vi "End experiment.vi"(7 "API Key":string, 8 "error in":errorcluster, 11 "Experiment ID":i32) -> (0 "error out":errorcluster)   [LabVIEW 2018]
uses:
  <vilib>/httpClient/PUTBuffer.vi
  <vilib>/httpClient/LabVIEWHTTPClient.lvlib
panel:
  out "Ended at response":string
  out "Server response debug panel":string
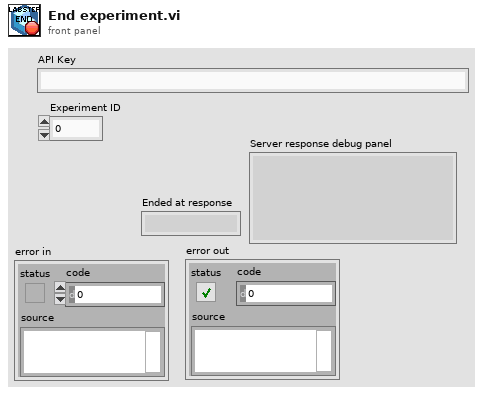
[diagram p1: front panel]
types:
  T1 = typedef "LabVIEWHTTPClient.lvlib/ClientHandle.ctl" = refnum<k1>
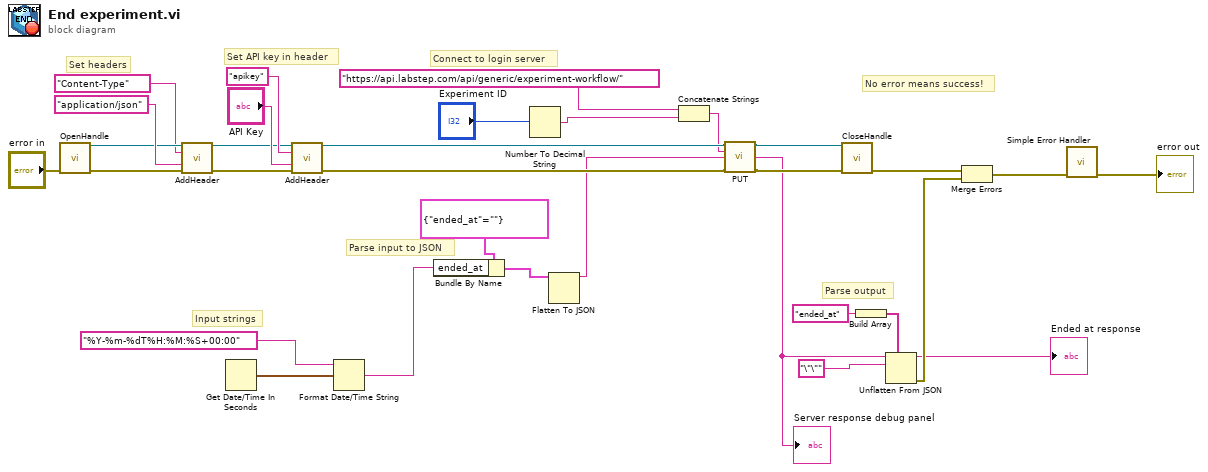
[diagram p0: block diagram]
diagram:
  # "No error means success!"
  # "Parse output"
  # "Set API key in header"
  # "Input strings"
  # "Set headers"
  # "Connect to login server"
  # "Parse input to JSON"
  n1 = call <vilib>:"OpenHandle.vi"("error in (no error)"="error in") -> ("client handle out"=w31:T1, "error out"=w30:errorcluster)  [unwired: 13 in]
  n2 = call <vilib>:"AddHeader.vi"("client handle"=w31, "header"="Content-Type", "value"="application/json", "error in (no error)"=w30) -> ("client handle out"=w22:T1, "error out"=w23:errorcluster)  [unwired: 10 in]
  n3 = Get Date/Time In Seconds() -> (seconds since 1Jan1904=w13:timestamp)
  n4 = call <vilib>:"AddHeader.vi"("client handle"=w22, "header"="apikey", "value"="API Key", "error in (no error)"=w23) -> ("client handle out"=w8:T1, "error out"=w7:errorcluster)  [unwired: 10 in]
  n5 = Format Date/Time String(time format string (%c)="%Y-%m-%dT%H:%M:%S+00:00", seconds (now)=w13) -> (date/time string=w11:string)  [unwired: 1 in]
  n6 = Bundle By Name(cluster=cluster{"ended_at":string} {"ended_at"=""}, "ended_at"=w11) -> (w29:cluster{"ended_at":string})
  n7 = Number To Decimal String(number="Experiment ID") -> (decimal integer string=w2:string)  [unwired: 1 in]
  n8 = Flatten To JSON(anything=w29) -> (JSON string=w6:string)  [unwired: 2 in, 1 out]
  n9 = Concatenate Strings("https://api.labstep.com/api/generic/experiment-workflow/" ("url"), w2) -> (w4:string)
  n10 = call-poly <vilib>:"PUT.vi"("client handle"=w8, "url"=w4, "buffer"=w6, "error in (no error)"=w7) -> ("client handle out"=w9:T1, "body"=w3:string, "error out"=w10:errorcluster)  [unwired: 8 in, 1 out]
  "Server response debug panel" <- w3
  n11 = call <vilib>:"CloseHandle.vi"("client handle"=w9, "error in (no error)"=w10) -> ("error out"=w16:errorcluster)  [unwired: 13 in]
  n12 = Build Array("ended_at") -> (w19:string[])
  n13 = Unflatten From JSON(path=w19, JSON string=w3, type and defaults="\"\"") -> (value=→"Ended at response":string, error out=w15:errorcluster)  [unwired: 4 in]
  n14 = Merge Errors(w16, w15) -> (w18:errorcluster)
  n15 = call <vilib>:"Simple Error Handler.vi"("error in (no error)"=w18) -> ("error out"=→"error out":errorcluster)  [unwired: 4 in, 4 out]
